vi "onProcessStartedWithErrors.vi"(8 "error in (no error)":errorcluster, 10 "Start error":errorcluster, 11 "MeasuringDevice":refnum<class "MeasuringDevice.lvclass">) -> (0 "error out":errorcluster, 3 "MeasuringDevice out":refnum<class "MeasuringDevice.lvclass">)   [LabVIEW 2017, in "MeasuringDevice.lvclass"]
doc: "JKI State Machine Objects (SMO) 1.3.0.56\nJKI - JKI\nCopyright (c) 2017, JKI"
uses:
  MeasuringDevice.lvclass
  <vilib>/JKI/JKI SMO/SMO/SMO.lvclass
panel:
  # "For instructions on how to use the JKI State Machine Objects, examples and video tutorials, visit:\nhttp://jki.net/state-machine-objects/\n\nJKI State Machine Objects™\nhttp://jki.net/state-machine-objects/\nCopyright (C) 2005-2015, JKI <info@jki.net>\nALL RIGHTS RESERVED"
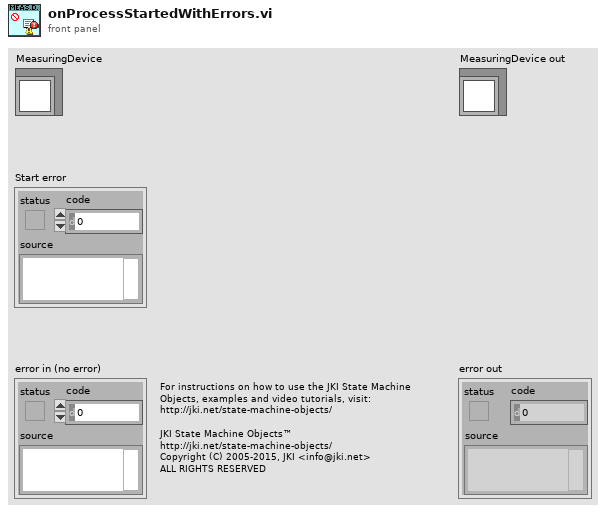
[diagram p1: front panel]
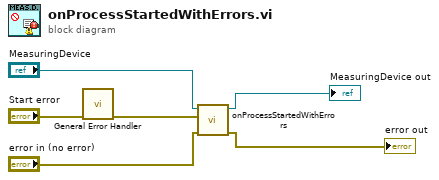
[diagram p0: block diagram]
diagram:
  n1 = call <vilib>:"General Error Handler.vi"("error in (no error)"="Start error") -> ("error out"=w3:errorcluster)  [unwired: 10 in, 4 out]
  n2 = call-parent "onProcessStartedWithErrors.vi"("error in (no error)"="error in (no error)", "Start error"=w3, "SMO"="MeasuringDevice") -> ("error out"=→"error out":errorcluster, "SMO out"=→"MeasuringDevice out":refnum<class "MeasuringDevice.lvclass">)  [unwired: 7 in]
